vi "Vector3DMagnitude.vi"(10 "Vector3D":T1) -> (2 "Magnitude":dbl)   [LabVIEW 2018]
uses:
  Vector3D.ctl
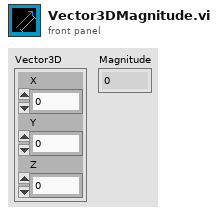
[diagram p1: front panel]
types:
  T1 = typedef "Vector3D.ctl" = cluster{"X":dbl, "Y":dbl, "Z":dbl}
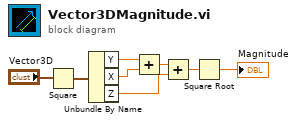
[diagram p0: block diagram]
diagram:
  n1 = Square(x="Vector3D") -> (x^2=w7:T1)
  n2 = Unbundle By Name(w7) -> ("Y"=w5:dbl, "X"=w4:dbl, "Z"=w3:dbl)
  n3 = Add(x=w5, y=w4) -> (x+y=w2:dbl)
  n4 = Add(x=w2, y=w3) -> (x+y=w1:dbl)
  n5 = Square Root(x=w1) -> (sqrt(x)=→"Magnitude":dbl)
